vi "LoadNodeUIStandardEvents.vi"(7 "Standard Event":T1, 8 "error in":errorcluster, 9 "sub panel ref":refnum<vi>, 10 "main queue":T8, 11 "node":T7) -> (0 "error out":errorcluster)   [LabVIEW 2025, in "CEF.lvlib"]
doc: "This VI will insert the UI from a node into a subpanel. Copyright 2017 National Instruments Corporation\n\nLicensed under the Apache License, Version 2.0 (the \"License\"); you may not use this file except in compliance with the License. You may obtain a copy of the License at http://www.apache.org/licenses/LICENSE-2.0\nUnless required by applicable law or agreed to in writing, software distributed under the License is distributed on an \"AS IS\" BASIS, WITHOUT WARRANTIES OR CONDITIONS OF ANY KIND, either express or implied. See the License for the specific language governing permissions and limitations under the License."
uses:
  CEF.lvlib
  Node/mainQref.ctl
  Node/NodeRef.ctl
  Node/CEF_Node.lvclass
  Node/StandardEvents.ctl
  Node/UserEventRef.ctl
  Controls/EventCluster.ctl
  Node/NodeChangeEvent.ctl
  Node/CacheState.ctl
  Node/RefreshUIEvent.ctl
  Node/StopEvent.ctl
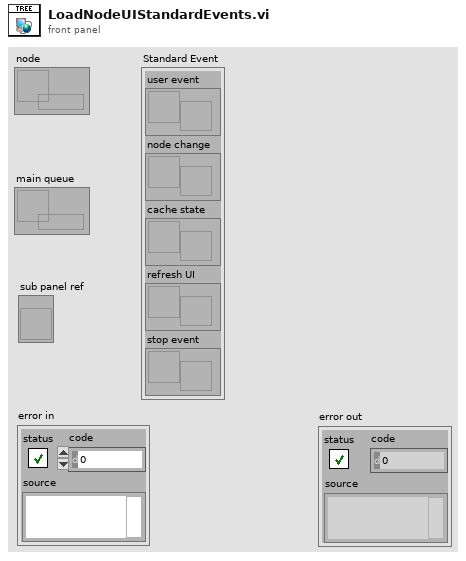
[diagram p1: front panel]
types:
  T1 = typedef "CEF.lvlib/CEF_Node.lvclass/StandardEvents.ctl" = cluster{"user event":T2, "node change":T3, "cache state":T4, "refresh UI":T5, "stop event":T6}
  T2 = typedef "CEF.lvlib/CEF_Node.lvclass/UserEventRef.ctl" = refnum<user-event>
  T3 = typedef "CEF.lvlib/CEF_Node.lvclass/NodeChangeEvent.ctl" = refnum<user-event>
  T4 = typedef "CEF.lvlib/CEF_Node.lvclass/CacheState.ctl" = refnum<user-event>
  T5 = typedef "CEF.lvlib/CEF_Node.lvclass/RefreshUIEvent.ctl" = refnum<user-event>
  T6 = typedef "CEF.lvlib/CEF_Node.lvclass/StopEvent.ctl" = refnum<user-event>
  T7 = typedef "CEF.lvlib/CEF_Node.lvclass/NodeRef.ctl" = refnum<data-value>
  T8 = typedef "CEF.lvlib/CEF_Node.lvclass/mainQref.ctl" = refnum<queue>
  T9 = enum32{"Bad", "Idle", "Run top level", "Running"}
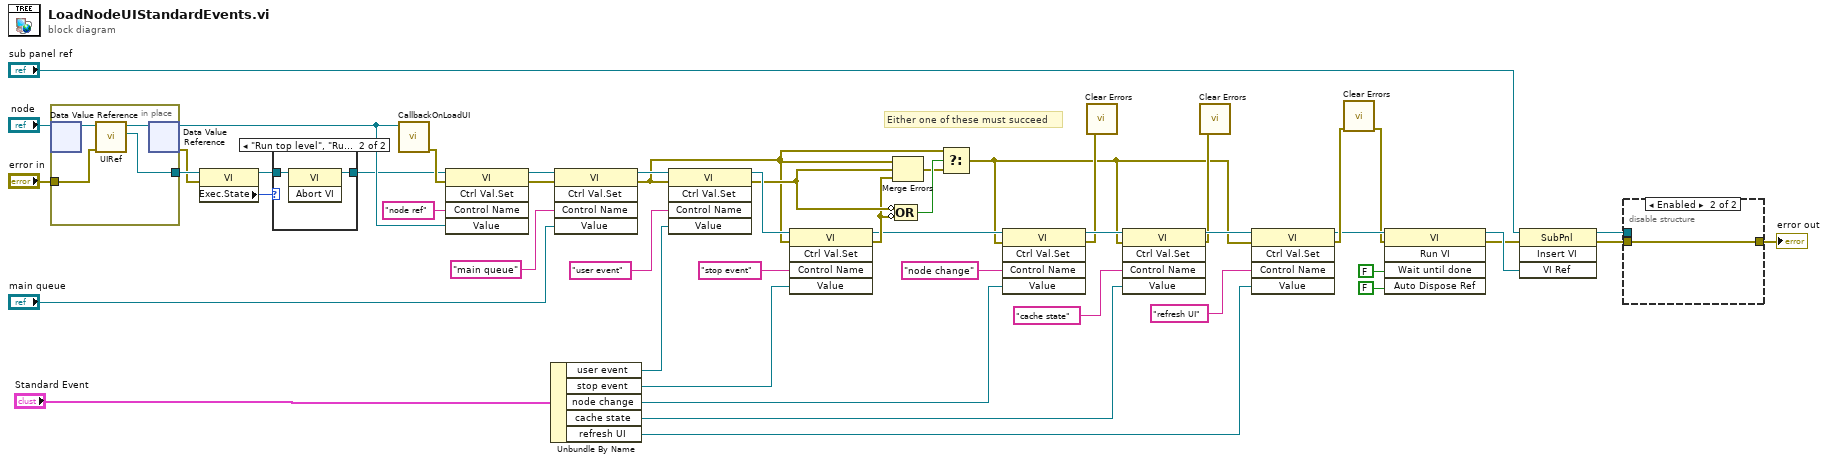
[diagram p0: block diagram]
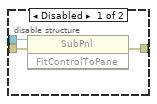
[diagram p2: hidden frame]
diagram:
  # "Either one of these must succeed"
  n1 = in-place {
    in-place-border: [w51] -> w11
    in-place-border: "error in" -> [w50]
    n2 = in-place-dvr #1("node") -> (w53:refnum<class "CEF_Node.lvclass">)  [unwired: 1 out]
    n3 = call-dynamic "UIRef.vi"("error in"=w50, 11:w53) -> ("VI refnum"=w51:refnum<vi>, "CEF_Node out"=w52:refnum<class "CEF_Node.lvclass">)  [unwired: 7 in, 1 out]
    n4 = in-place-dvr #1(w52) -> (w21:T7, w6:errorcluster)
  }
  n5 = property class="VI"(reference=w11, error in=w6) -> (reference out=w9:refnum<vi>, "Exec.State"=w10:T9)  [unwired: 1 out]
  n6 = case shown="\"Run top level\", \"Running\"" w10 {
    tunnel: w9 -> [w54 w56]
    tunnel: [w54 w55] -> w8
    frame "Idle", Default {
    }
    frame "Run top level", "Running" {
      n7 = invoke class="VI" method="Abort VI"(reference=w56) -> (reference out=w55:refnum<vi>)  [unwired: 2 in, 2 out]
    }
  }
  n8 = call "CallbackOnLoadUI.vi"("node"=w21) -> ("error out"=w22:errorcluster)  [unwired: 10 in]
  n9 = invoke class="VI" method="Ctrl Val.Set"(reference=w8, error in=w22, "Control Name"="node ref", "Value"=w21) -> (reference out=w44:refnum<vi>, error out=w43:errorcluster)  [unwired: 1 in, 3 out]
  n10 = Unbundle By Name("Standard Event") -> ("user event"=w40:T2, "stop event"=w38:T6, "node change"=w25:T3, "cache state"=w24:T4, "refresh UI"=w23:T5)
  n11 = invoke class="VI" method="Ctrl Val.Set"(reference=w44, error in=w43, "Control Name"="main queue", "Value"="main queue") -> (reference out=w42:refnum<vi>, error out=w32:errorcluster)  [unwired: 1 in, 3 out]
  n12 = invoke class="VI" method="Ctrl Val.Set"(reference=w42, error in=w32, "Control Name"="user event", "Value"=w40) -> (reference out=w39:refnum<vi>, error out=w36:errorcluster)  [unwired: 1 in, 3 out]
  n13 = invoke class="VI" method="Ctrl Val.Set"(reference=w39, error in=w32, "Control Name"="stop event", "Value"=w38) -> (reference out=w31:refnum<vi>, error out=w35:errorcluster)  [unwired: 1 in, 3 out]
  n14 = Merge Errors(w32, w36, w35) -> (w33:errorcluster)
  n15 = Compound Arithmetic op=OR(invert w36, invert w35) -> (w34:bool)
  n16 = Select(t=w32, s=w34, f=w33) -> (s? t:f=w2:errorcluster)
  n17 = invoke class="VI" method="Ctrl Val.Set"(reference=w31, error in=w2, "Control Name"="node change", "Value"=w25) -> (reference out=w30:refnum<vi>, error out=w17:errorcluster)  [unwired: 1 in, 3 out]
  n18 = call <vilib>:"Clear Errors.vi"("error in (no error)"=w17) -> ()  [unwired: 5 in, 2 out]
  n19 = invoke class="VI" method="Ctrl Val.Set"(reference=w30, error in=w2, "Control Name"="cache state", "Value"=w24) -> (reference out=w29:refnum<vi>, error out=w16:errorcluster)  [unwired: 1 in, 3 out]
  n20 = call <vilib>:"Clear Errors.vi"("error in (no error)"=w16) -> ()  [unwired: 5 in, 2 out]
  n21 = invoke class="VI" method="Ctrl Val.Set"(reference=w29, error in=w2, "Control Name"="refresh UI", "Value"=w23) -> (reference out=w12:refnum<vi>, error out=w15:errorcluster)  [unwired: 1 in, 3 out]
  n22 = call <vilib>:"Clear Errors.vi"("error in (no error)"=w15) -> ("error out"=w1:errorcluster)  [unwired: 5 in, 1 out]
  n23 = invoke class="VI" method="Run VI"(reference=w12, error in=w1, "Wait until done"=FALSE ("Wait Until Done"), "Auto Dispose Ref"=FALSE ("Auto Dispose Reference")) -> (reference out=w19:refnum<vi>, error out=w18:errorcluster)  [unwired: 1 in, 3 out]
  n24 = invoke class="SubPnl" method="Insert VI"(reference="sub panel ref", error in=w18, "VI Ref"=w19) -> (reference out=w5:refnum<vi>, error out=w4:errorcluster)  [unwired: 1 in, 2 out]
  n25 = disable-structure shown="Enabled" {
    disable-tunnel: w5 -> [w59 _]
    disable-tunnel: w4 -> [w58 w60]
    disable-tunnel: [w57 w60] -> w3
    frame Disabled {
      n26 = invoke class="SubPnl" method="FitControlToPane"(reference=w59, error in=w58) -> (error out=w57:errorcluster)  [unwired: 1 in, 2 out]
    }
    frame Enabled {
    }
  }
  "error out" <- w3
